vi "tanqueexample.vi"() -> ()   [LabVIEW 2015]
panel:
  in  "Finalizar":bool
  in  "Abierto":bool
  in  "Disminuir":bool
  out "Tank":dbl(slide) scale=0.0..100.0
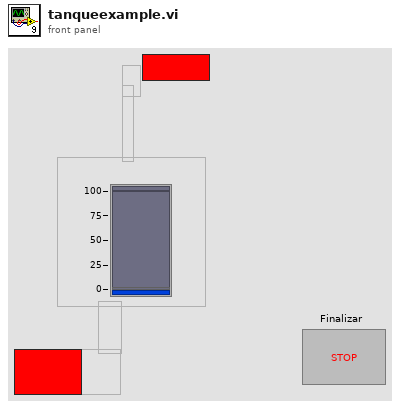
[diagram p1: front panel]
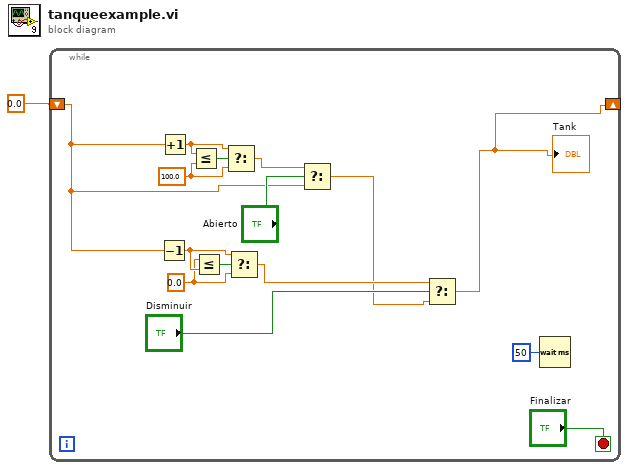
[diagram p0: block diagram]
diagram:
  n1 = while {
    shift-right: [w3] -> _
    shift-left: 0.0 -> [w5]
    stop <- "Finalizar" stop-if-true
    w10 = 100.0 ("y")
    w13 = 0.0 ("y")
    n2 = Decrement(x=w5) -> (x-1=w14:dbl)
    n3 = Increment(x=w5) -> (x+1=w11:dbl)
    n4 = Less Or Equal?(x=w11, y=w10) -> (x <= y?=w12:bool)
    n5 = Less Or Equal?(x=w13, y=w14) -> (x <= y?=w15:bool)
    n6 = Select(t=w11, s=w12, f=w10) -> (s? t:f=w8:dbl)
    n7 = Select(t=w14, s=w15, f=w13) -> (s? t:f=w6:dbl)
    n8 = Select(t=w8, s="Abierto", f=w5) -> (s? t:f=w4:dbl)
    n9 = Select(t=w6, s="Disminuir", f=w4) -> (s? t:f=w3:dbl)
    "Tank" <- w3
    n10 = Wait (ms)(milliseconds to wait=u32 50) -> ()  [unwired: 1 out]
  }
